vi "Init Control Value - Num.vi"(8 "error in (no error)":errorcluster, 10 "Num Control Names":string[](array[string]), 11 "This VI":refnum<vi>) -> (0 "error out":errorcluster, 2 "PLC IP":string, 3 "Config File Path":path)   [LabVIEW 2018]
uses:
  <vilib>/Utility/config.llb/Read Key (Double).vi
  <vilib>/Utility/config.llb/Write Key (Double).vi
  <vilib>/Utility/config.llb/Read Key (String).vi
  <vilib>/Utility/config.llb/Write Key (String).vi
  <vilib>/Utility/config.llb/NI_LVConfig.lvlib
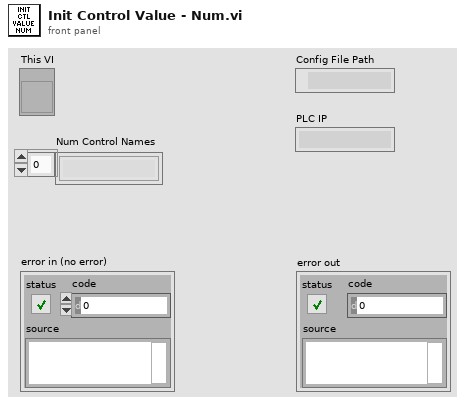
[diagram p1: front panel]
types:
  T1 = typedef "NI_LVConfig.lvlib/Config Data RefNum.ctl" = refnum<k1>
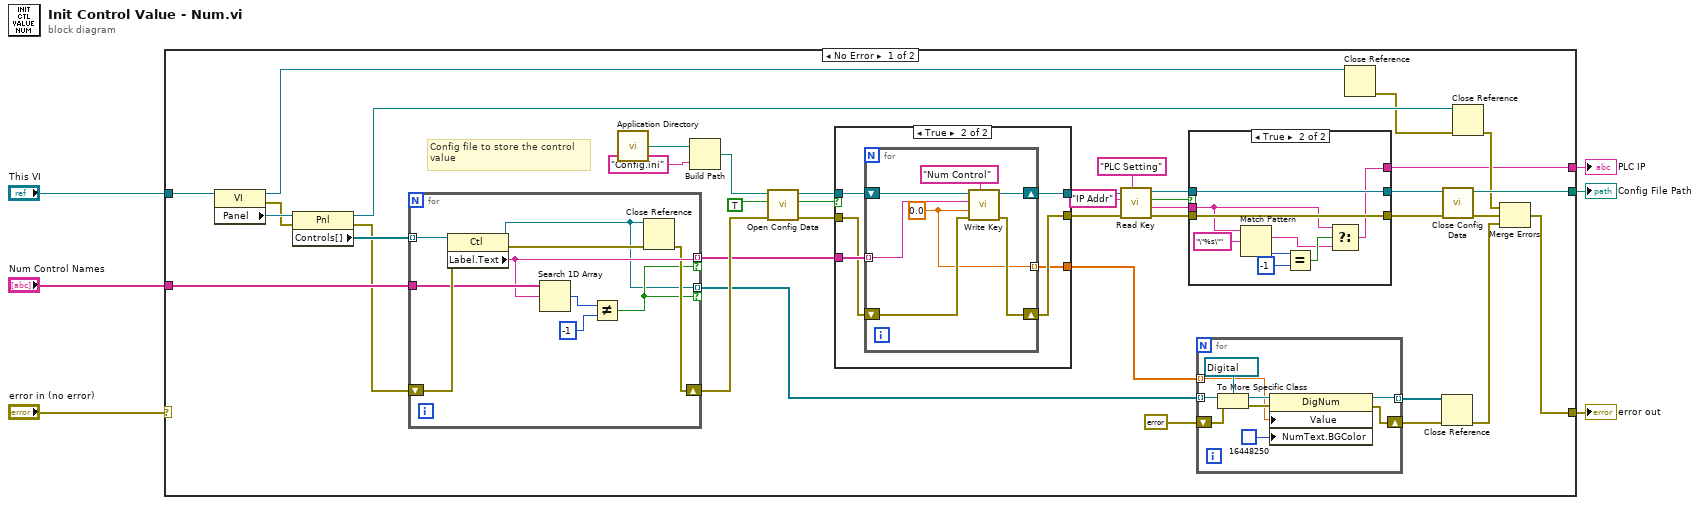
[diagram p0: block diagram]
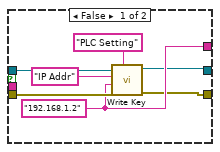
[diagram p2: hidden frame]
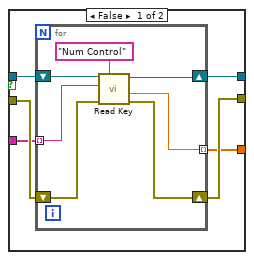
[diagram p3: hidden frame]
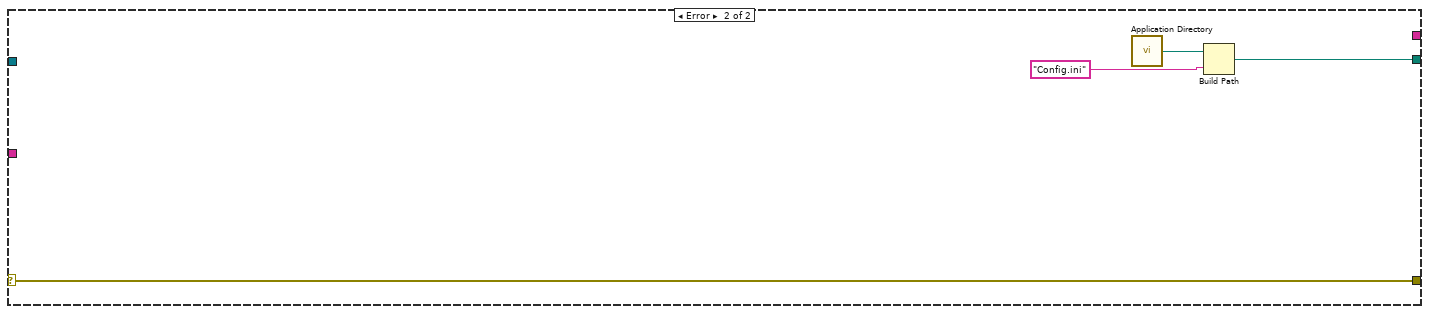
[diagram p4: hidden frame]
diagram:
  n1 = case shown="No Error" "error in (no error)" {
    selector: "error in (no error)" -> [_ w107]
    tunnel: "Num Control Names" -> [w42 _]
    tunnel: "This VI" -> [w43 _]
    tunnel: [w27 w108] -> w2
    tunnel: [w24 w107] -> w3
    tunnel: [w11 _] -> w1
    frame No Error {
      # "Config file to store the control\nvalue"
      n2 = property class="VI"(reference=w43) -> (reference out=w30:refnum<vi>, error out=w44:errorcluster, "Panel"=w45:refnum<vi>)  [unwired: 1 in]
      n3 = property class="Pnl"(reference=w45, error in=w44) -> (reference out=w29:refnum<vi>, error out=w40:errorcluster, "Controls[]"=w41:refnum<vi>[])
      n4 = for {
        tunnel: w41 -> [w106] mode=indexing
        shift-right: [w99] -> w38
        shift-left: w40 -> [w105]
        tunnel: w42 -> [w104]
        tunnel: [w101] -> w35 mode=indexing if=w98
        tunnel: [w97] -> w22 mode=indexing if=w98
        n5 = property class="Ctl"(reference=w106, error in=w105) -> (reference out=w97:refnum<vi>, error out=w100:errorcluster, "Label.Text"=w101:string)
        n6 = Search 1D Array(1D array=w104, element=w101) -> (index of element=w103:i32)  [unwired: 1 in]
        n7 = Not Equal?(x=w103, y=-1) -> (x != y?=w98:bool)
        n8 = Close Reference(reference=w97, error in (no error)=w100) -> (error out=w99:errorcluster)
      }
      n9 = call <vilib>:"Application Directory.vi"() -> ("Application Directory"=w33:path)
      n10 = Build Path(base path=w33, name or relative path="Config.ini") -> (appended path=w31:path)
      n11 = call <vilib>:"Open Config Data.vi"("error in (no error)"=w38, "create file if necessary (T)"=TRUE, "configuration file path"=w31) -> ("error out"=w34:errorcluster, "file created?"=w37:bool, "refnum"=w36:T1)  [unwired: 6 in]
      n12 = case shown="True" w37 {
        tunnel: w36 -> [w76 w88]
        tunnel: w35 -> [w74 w89]
        tunnel: w34 -> [w75 w87]
        tunnel: [w73 w86] -> w17
        tunnel: [w72 w85] -> w16
        tunnel: [w71 w84] -> w21
        frame False {
          n13 = for {
            shift-right: [w80] -> w73
            shift-left: w76 -> [w83]
            shift-right: [w78] -> w72
            shift-left: w75 -> [w81]
            tunnel: w74 -> [w79] mode=indexing
            tunnel: [w77] -> w71 mode=indexing
            n14 = call-poly <vilib>:"Read Key.vi"("section"="Num Control", "error in (no error)"=w81, "key"=w79, "refnum"=w83) -> ("error out"=w78:errorcluster, "value"=w77:dbl, "refnum out"=w80:T1)  [unwired: 4 in, 1 out]
          }
        }
        frame True {
          n15 = for {
            tunnel: w89 -> [w94] mode=indexing
            shift-right: [w92] -> w86
            shift-left: w88 -> [w95]
            shift-right: [w91] -> w85
            shift-left: w87 -> [w93]
            tunnel: [w90] -> w84 mode=indexing
            w90 = 0.0
            n16 = call-poly <vilib>:"Write Key.vi"("section"="Num Control", "error in (no error)"=w93, "value"=w90, "key"=w94, "refnum"=w95) -> ("error out"=w91:errorcluster, "refnum out"=w92:T1)  [unwired: 3 in, 2 out]
          }
        }
      }
      n17 = call-poly <vilib>:"Read Key.vi"("section"="PLC Setting", "error in (no error)"=w16, "key"="IP Addr", "refnum"=w17) -> ("error out"=w8:errorcluster, "value"=w12:string, "found?"=w13:bool, "refnum out"=w10:T1)  [unwired: 4 in]
      n18 = case shown="True" w13 {
        tunnel: w12 -> [_ w55]
        tunnel: [w48 w53] -> w11
        tunnel: w10 -> [w51 w61]
        tunnel: [w47 w61] -> w9
        tunnel: w8 -> [w50 w60]
        tunnel: [w46 w60] -> w7
        frame False {
          w48 = "192.168.1.2" ("key")
          n19 = call-poly <vilib>:"Write Key.vi"("section"="PLC Setting", "error in (no error)"=w50, "value"=w48, "key"="IP Addr", "refnum"=w51) -> ("error out"=w46:errorcluster, "refnum out"=w47:T1)  [unwired: 1 in, 4 out]
        }
        frame True {
          n20 = Match Pattern(string=w55, regular expression="\"%s\"") -> (match substring=w54:string, offset past match=w58:i32)  [unwired: 1 in, 2 out]
          n21 = Equal?(x=w58, y=-1) -> (x = y?=w56:bool)
          n22 = Select(t=w55, s=w56, f=w54) -> (s? t:f=w53:string)
        }
      }
      n23 = for {
        tunnel: w22 -> [w66] mode=indexing
        shift-right: [w63] -> w18
        shift-left: errorcluster {"status"=FALSE, "code"=0, "source"=""} ("error constant") -> [w65]
        tunnel: w21 -> [w64] mode=indexing
        tunnel: [w62] -> w20 mode=indexing
        n24 = To More Specific Class(target class=refnum<vi> refnum ("Numeric"), reference=w66, error in=w65) -> (specific class reference=w69:refnum<vi>, error out=w70:errorcluster)
        n25 = property class="DigNum"(reference=w69, error in=w70, "Value"=w64, "NumText.BGColor"=u32 16448250) -> (reference out=w62:refnum<vi>, error out=w63:errorcluster)
      }
      n26 = Close Reference(reference=w30) -> (error out=w28:errorcluster)  [unwired: 1 in]
      n27 = Close Reference(reference=w20, error in (no error)=w18) -> (error out=w23:errorcluster)
      n28 = call <vilib>:"Close Config Data.vi"("error in (no error)"=w7, "refnum"=w9) -> ("error out"=w25:errorcluster, "file path"=w27:path)  [unwired: 8 in]
      n29 = Close Reference(reference=w29, error in (no error)=w28) -> (error out=w26:errorcluster)
      n30 = Merge Errors(w26, w25, w23) -> (w24:errorcluster)
    }
    frame Error {
      n31 = call <vilib>:"Application Directory.vi"() -> ("Application Directory"=w110:path)
      n32 = Build Path(base path=w110, name or relative path="Config.ini") -> (appended path=w108:path)
    }
  }
  "error out" <- w3
  "Config File Path" <- w2
  "PLC IP" <- w1
